vi "Get Resource Type.vi"(11 "AnalogIn in":refnum<class "AnalogIn.lvclass">) -> (2 "Resource Type":string)   [LabVIEW 2020, in "CTI.lvlib" / "AnalogIn.lvclass"]
uses:
  AnalogIn.lvclass
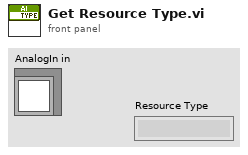
[diagram p1: front panel]
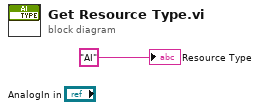
[diagram p0: block diagram]
diagram:
  "Resource Type" <- "AI" ("Resource Type")
